vi "Actor Core.vi"(8 "error in":errorcluster, 11 "Generador de Funciones in":refnum<class "Generador de Funciones.lvclass">) -> (0 "error out":errorcluster, 3 "Actor out":refnum<class "Actor.lvclass">)   [LabVIEW 2020, in "Generador de Funciones.lvlib" / "Generador de Funciones.lvclass"]
doc: "(<B>Filename</B>: Actor Framework.lvlib:Actor.lvclass:Actor Core.vi)\n\nReceives messages to the actor, reacts to them, and initiates any error handling that may shut the actor down.\n\nDescendant classes may override this VI to append parallel tasks for the actor to complete while it handles messages. Overrides use the Call Parent Class Method node."
uses:
  Generador de Funciones.lvclass
  C:/Program Files (x86)/National Instruments/LabVIEW 2020/vi.lib/ActorFramework/Actor/Actor.lvclass
  <vilib>/ActorFramework/Actor/Actor.lvclass
  Loggin/Loggin/Loggin.lvclass
  Generador de Funciones.lvclass/Generador de Funciones.ctl
  <vilib>/ActorFramework/Actor/Actor.lvclass/Actor.ctl
  <vilib>/ActorFramework/Message Enqueuer/Message Enqueuer.lvclass/Message Enqueuer.ctl
  Loggin/Loggin Messages/saveDAta Msg/saveDAta Msg.lvclass/saveDAta Msg.ctl
  <vilib>/ActorFramework/Message Enqueuer/Enqueue.vi
  <vilib>/ActorFramework/Stop Msg/Stop Msg.lvclass
  C:/Program Files (x86)/National Instruments/LabVIEW 2020/vi.lib/ActorFramework/Message/Message.lvclass
  Loggin/Loggin Messages/saveDAta Msg/saveDAta Msg.lvclass
  <vilib>/ActorFramework/Message Priority Queue/Priority Enqueue.vi
panel:
  in  "Guardar Parametros":cluster{"Tipo de archivo":u16, "File Path":path} {"Tipo de archivo" items=["Texto plano", "TDMS"]}
  in  "Parametros de la señal":T1
  in  "Save Button":bool
  in  "Stop":bool
  in  "Start":bool
  out "Waveform Chart":waveform(dbl)(graph)
  in  "Exit":bool
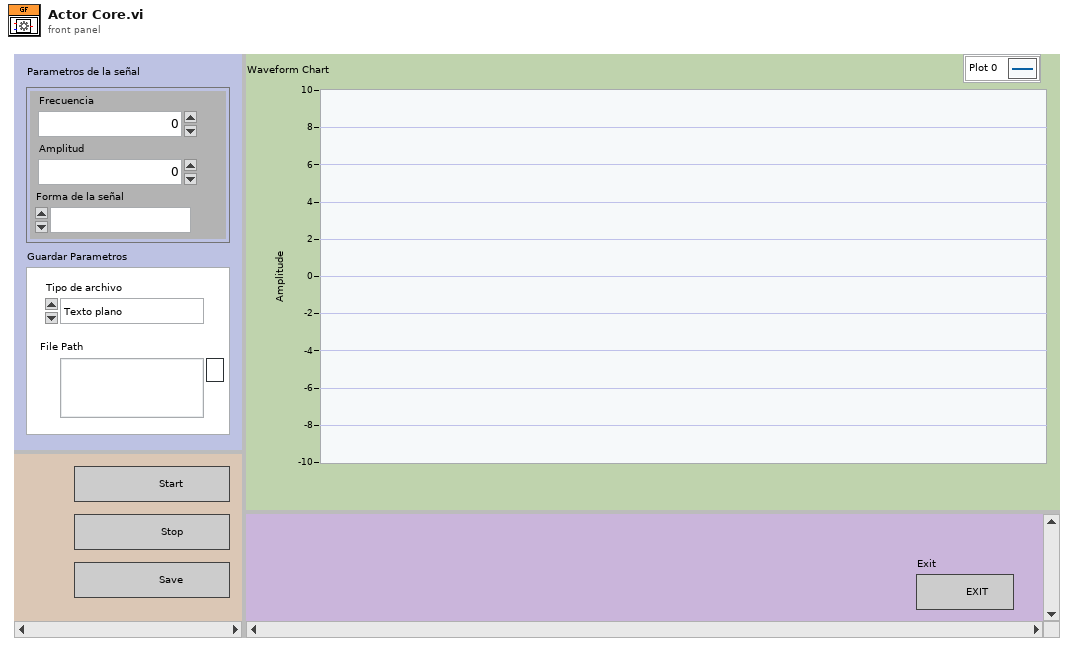
[diagram p1: front panel]
types:
  T1 = cluster{"Frecuencia":dbl, "Amplitud":dbl, "Forma de la señal":u16}
  T2 = cluster{"Generar Señal Event":refnum<user-event>, "Event stop":refnum<user-event>}
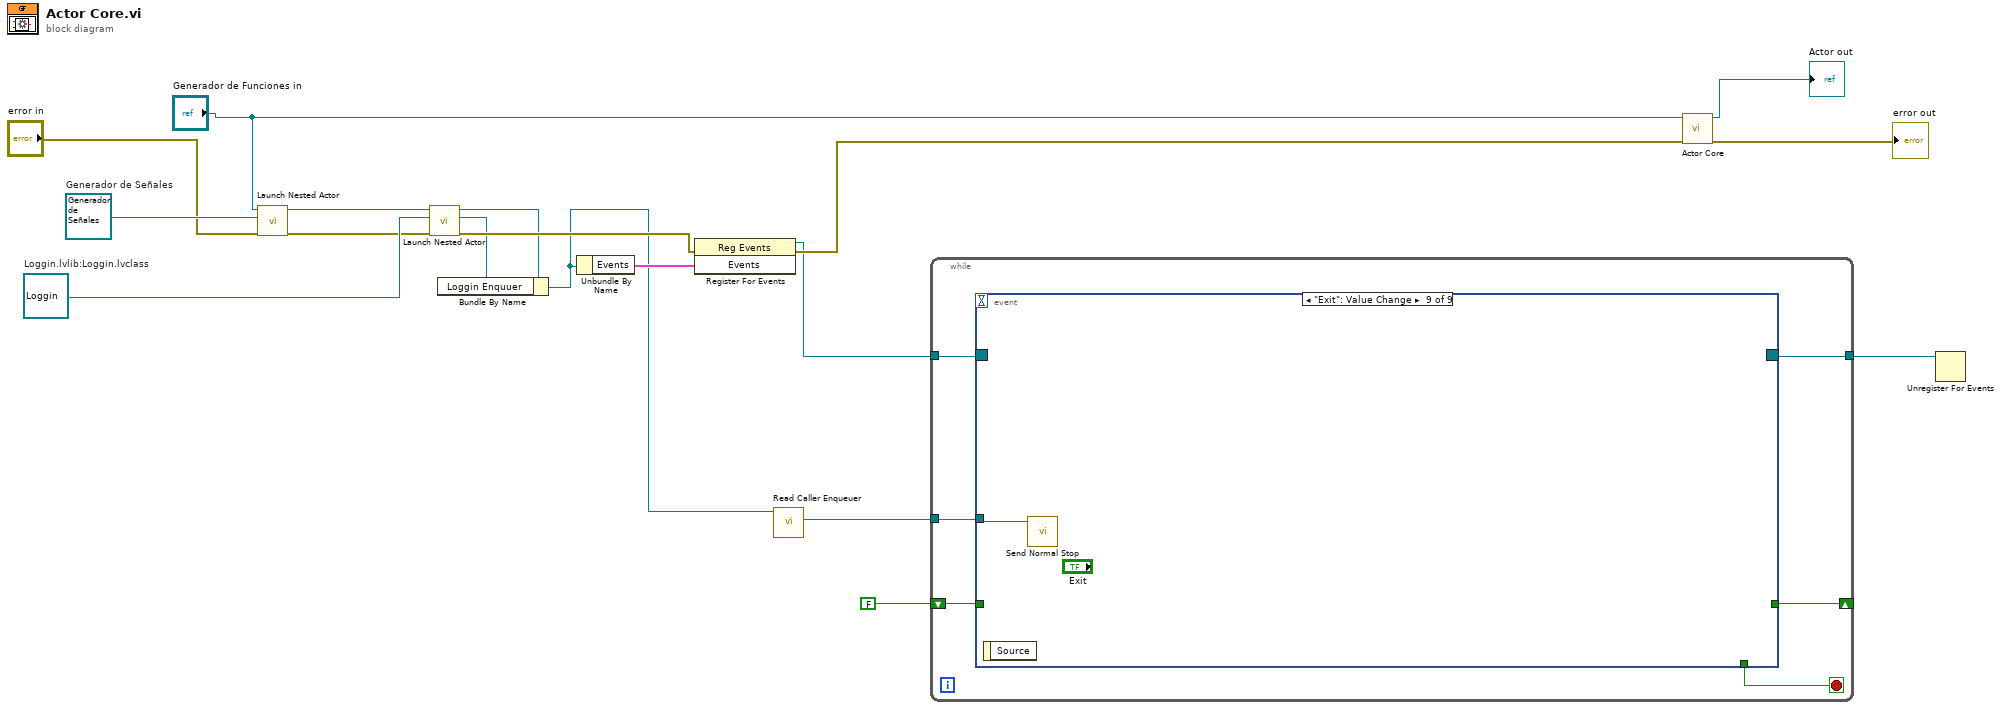
[diagram p0: block diagram]
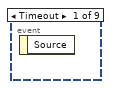
[diagram p2: hidden frame]
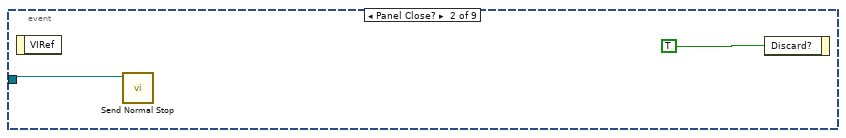
[diagram p3: hidden frame]
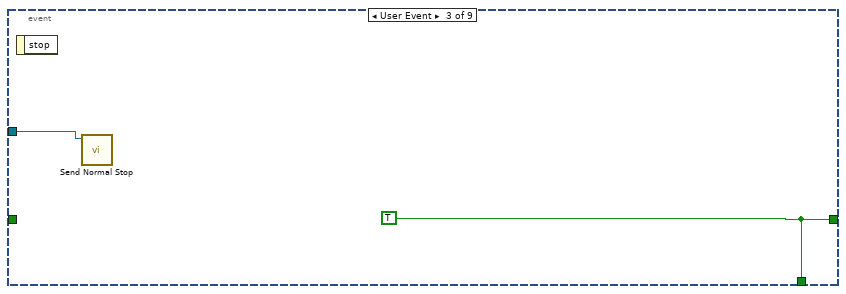
[diagram p4: hidden frame]
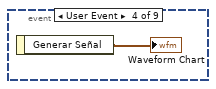
[diagram p5: hidden frame]
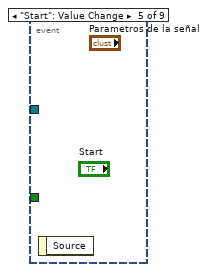
[diagram p6: hidden frame]
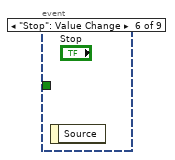
[diagram p7: hidden frame]
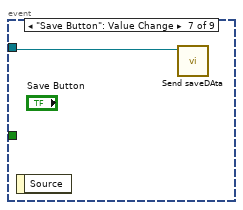
[diagram p8: hidden frame]
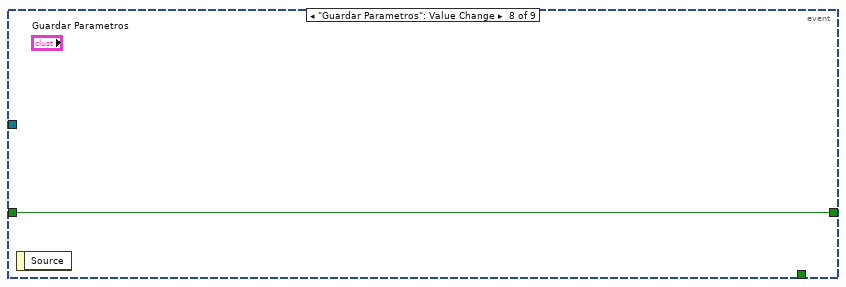
[diagram p9: hidden frame]
diagram:
  w7 = refnum<class "Loggin.lvclass"> refnum  # Loggin.lvlib:Loggin.lvclass
  w14 = refnum<class "Generador de Señales.lvclass"> refnum  # Generador de Señales
  n1 = call <vilib>:"Launch Nested Actor.vi"("error in (no error)"="error in", "Nested Actor"=w14, "Caller Actor in"="Generador de Funciones in") -> ("error out"=w5:errorcluster, "Caller Actor out"=w8:refnum<class "Generador de Funciones.lvclass">)  [unwired: 6 in, 1 out]
  n2 = call <vilib>:"Launch Nested Actor.vi"("error in (no error)"=w5, "Nested Actor"=w7, "Caller Actor in"=w8) -> ("error out"=w4:errorcluster, "Nested Actor's Enqueuer"=w1:refnum<class "Message Enqueuer.lvclass">, "Caller Actor out"=w3:refnum<class "Generador de Funciones.lvclass">)  [unwired: 6 in]
  n3 = Bundle By Name(cluster=w3, "Loggin Enquuer"=w1) -> (w2:refnum<class "Generador de Funciones.lvclass">)
  n4 = Unbundle By Name(w2) -> ("Events"=w12:T2)
  n5 = register-events(error in=w4, w12) -> (reference out=w10:refnum<event-registration>, error out=w11:errorcluster)  [unwired: 1 in]
  n6 = call <vilib>:"Read Caller Enqueuer.vi"("Actor"=w2) -> ("Caller Enqueuer"=w9:refnum<class "Message Enqueuer.lvclass">)  [unwired: 10 in]
  n7 = while {
    shift-right: [w23] -> _
    shift-left: FALSE -> [w24]
    tunnel: [w22] -> w15
    tunnel: w10 -> [w21]
    tunnel: w9 -> [w20]
    stop <- w19 stop-if-true
    n8 = event shown="[8] \"Exit\": Value Change" {
      selector: w21 -> [_ _ _ _ _ _ _ _ _]
      dyn-events: [_ _ _ _ _ _ _ _ _] -> w22
      timeout: _ -> [_ _ _ _ _ _ _ _ _]
      tunnel: w24 -> [_ _ _ _ _ _ _ w31 _]
      tunnel: [_ _ w27 _ _ _ _ w31 _] -> w23
      tunnel: w20 -> [_ w25 w28 _ _ _ w30 _ w32]
      tunnel: [_ _ w27 _ _ _ _ _ _] -> w19
      event Timeout {
        n9 = event-data() -> ()  [unwired: 1 in, 1 out]
      }
      event Panel Close? {
        n10 = event-data() -> ()  [unwired: 1 in, 1 out]
        n11 = call <vilib>:"Send Normal Stop.vi"("Message Enqueuer"=w25) -> ()  [unwired: 10 in, 1 out]
        n12 = event-data("Discard?"=TRUE) -> ()  [unwired: 1 in, 1 out]
      }
      event User Event {
        w27 = TRUE
        n13 = event-data() -> ()  [unwired: 1 in, 1 out]
        n14 = call <vilib>:"Send Normal Stop.vi"("Message Enqueuer"=w28) -> ()  [unwired: 10 in, 1 out]
      }
      event User Event {
        n15 = event-data() -> ("Generar Señal"=→"Waveform Chart":waveform(dbl))  [unwired: 1 in]
      }
      event "Start": Value Change {
        n16 = event-data() -> ()  [unwired: 1 in, 1 out]
      }
      event "Stop": Value Change {
        n17 = event-data() -> ()  [unwired: 1 in, 1 out]
      }
      event "Save Button": Value Change {
        n18 = event-data() -> ()  [unwired: 1 in, 1 out]
        n19 = call "Send saveDAta.vi"("Message Enqueuer"=w30) -> ()  [unwired: 9 in, 2 out]
      }
      event "Guardar Parametros": Value Change {
        n20 = event-data() -> ()  [unwired: 1 in, 1 out]
      }
      event "Exit": Value Change {
        n21 = event-data() -> ()  [unwired: 1 in, 1 out]
        n22 = call <vilib>:"Send Normal Stop.vi"("Message Enqueuer"=w32) -> ()  [unwired: 10 in, 1 out]
      }
    }
  }
  n23 = call-parent "Actor Core.vi"("error in"=w11, "Actor in"="Generador de Funciones in") -> ("error out"=→"error out":errorcluster, "Actor out"=→"Actor out":refnum<class "Actor.lvclass">)  [unwired: 8 in]
  n24 = Unregister For Events(event registration refnum=w15) -> ()  [unwired: 1 in, 1 out]
